vi "Set-Limits.vi"(2 "Minimum / V":dbl=-1.0 min=-15.0 max=15.0, 3 "Maximum / V":dbl=1.0 min=-15.0 max=15.0, 4 "error in (no error)":errorcluster, 6 "Output channel":T1, 7 "VISA resource name":refnum<visa-resource-name>="COM7") -> (0 "error out":errorcluster={"status"=TRUE, "code"=10, "source"="Setting the limits failed: return values not echoed correctly."}, 1 "VISA resource name out":refnum<visa-resource-name>="COM7")   [LabVIEW 2015, in "YbTempCtrl.lvlib"]
doc: "Set software limits for the maximum / minimum control signal"
uses:
  YbTempCtrl.lvlib
  Typedefs/OutputChannelTypedef.ctl
panel:
  out "Returned String":string
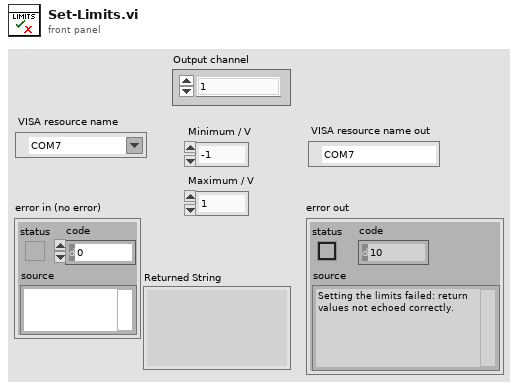
[diagram p1: front panel]
types:
  T1 = typedef "YbTempCtrl.lvlib/OutputChannelTypedef.ctl" = enum16{"1", "2", "3", "4", "BPA", "BPB"}
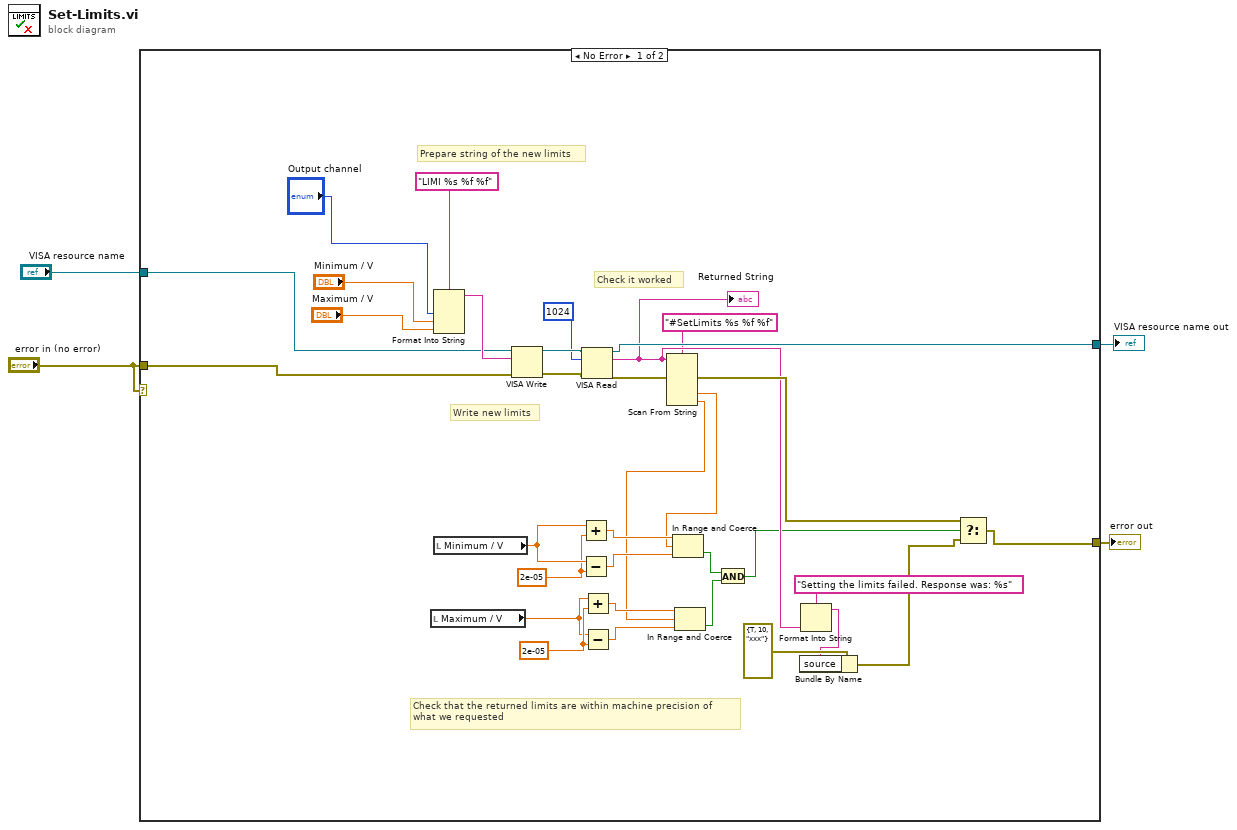
[diagram p0: block diagram]
diagram:
  n1 = case shown="No Error" "error in (no error)" {
    tunnel: "VISA resource name" -> [w14 w38]
    tunnel: "error in (no error)" -> [w13 w39]
    tunnel: [w20 w38] -> w3
    tunnel: [w19 w39] -> w2
    frame No Error {
      w26 = 2e-05
      w34 = 2e-05
      # "Check that the returned limits are within machine precision of\nwhat we requested"
      # "Check it worked"
      # "Write new limits"
      # "Prepare string of the new limits"
      n2 = local read "Maximum / V"() -> (w23:dbl)
      n3 = Format Into String(format string="LIMI %s %f %f", "Output channel", "Minimum / V", "Maximum / V") -> (resulting string=w36:string)  [unwired: 2 in, 1 out]
      n4 = local read "Minimum / V"() -> (w35:dbl)
      n5 = VISA Write(VISA resource name=w14, write buffer=w36, error in (no error)=w13) -> (VISA resource name out=w31:refnum<visa-resource-name>, error out=w30:errorcluster)  [unwired: 1 out]
      n6 = Add(x=w35, y=w34) -> (x+y=w33:dbl)
      n7 = Subtract(x=w35, y=w34) -> (x-y=w32:dbl)
      n8 = VISA Read(VISA resource name=w31, byte count=u32 1024, error in (no error)=w30) -> (VISA resource name out=w20:refnum<visa-resource-name>, read buffer=w8:string, error out=w28:errorcluster)  [unwired: 1 out]
      "Returned String" <- w8
      n9 = Add(x=w23, y=w26) -> (x+y=w25:dbl)
      n10 = Subtract(x=w23, y=w26) -> (x-y=w24:dbl)
      n11 = Scan From String(format string="#SetLimits %s %f %f", input string=w8, error in=w28) -> (error out=w27:errorcluster, output 2=w16:dbl, output 3=w15:dbl)  [unwired: 5 in, 2 out]
      n12 = In Range and Coerce(upper limit=w33, x=w16, lower limit=w32) -> (In Range?=w22:bool)  [unwired: 1 out]
      n13 = In Range and Coerce(upper limit=w25, x=w15, lower limit=w24) -> (In Range?=w21:bool)  [unwired: 1 out]
      n14 = And(x=w22, y=w21) -> (x .and. y?=w5:bool)
      n15 = Format Into String(format string="Setting the limits failed. Response was: %s", w8) -> (resulting string=w9:string)  [unwired: 2 in, 1 out]
      n16 = Bundle By Name(cluster=errorcluster {"status"=TRUE, "code"=10, "source"="xxx"} ("f"), "source"=w9) -> (w11:errorcluster)
      n17 = Select(t=w27, s=w5, f=w11) -> (s? t:f=w19:errorcluster)
    }
    frame Error {
    }
  }
  "VISA resource name out" <- w3
  "error out" <- w2
